vi "Read Harmonics Measure Item.vi"(0 "VISA resource name":refnum<visa-resource-name>, 5 "Harmonics Item (2: V)":u16(ring)=2 items=["Sync", "VTHD", "V", "VCON", "ATHD", "A", "ACON", "PF", "W", "WCON", "Vdeg", "Adeg"], 11 "error in (no error)":errorcluster) -> (4 "VISA resource name out":refnum<visa-resource-name>, 6 "Data":sgl[](array[numeric]) format="%^.3e", 15 "error out":errorcluster)   [LabVIEW 2013, in "Yokogawa WT200 Series.lvlib"]
doc: "This VI reads harmonic datas from the WT200 Series.\n\nNote : It needs /HRM option."
uses:
  <instrlib>/Yokogawa WT200 Series/Yokogawa WT200 Series.lvlib
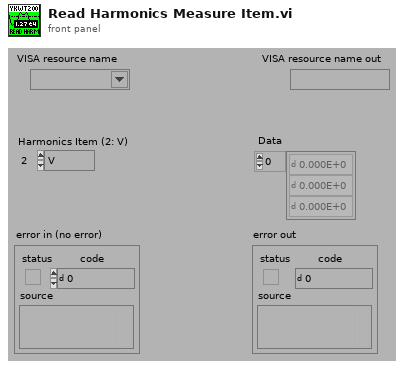
[diagram p1: front panel]
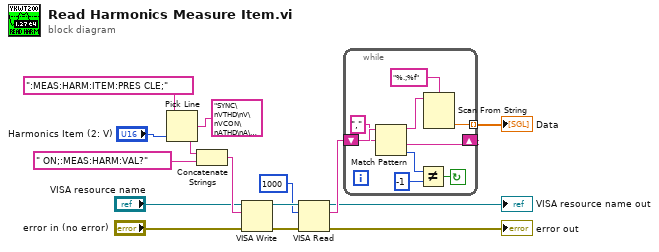
[diagram p0: block diagram]
diagram:
  n1 = Pick Line(string ("")=":MEAS:HARM:ITEM:PRES CLE;", multi-line string="SYNC\nVTHD\nV\nVCON\nATHD\nA\nACON\nPF\nW\nWCON\nVDEG\nADEG", line index="Harmonics Item (2: V)") -> (output string=w9:string)
  n2 = Concatenate Strings(w9, " ON;:MEAS:HARM:VAL?") -> (w7:string)
  n3 = VISA Write(VISA resource name="VISA resource name", write buffer=w7, error in (no error)="error in (no error)") -> (VISA resource name out=w14:refnum<visa-resource-name>, error out=w15:errorcluster)  [unwired: 1 out]
  n4 = VISA Read(VISA resource name=w14, byte count=u32 1000, error in (no error)=w15) -> (VISA resource name out=→"VISA resource name out":refnum<visa-resource-name>, read buffer=w6:string, error out=→"error out":errorcluster)  [unwired: 1 out]
  n5 = while {
    tunnel: [w17] -> w5 mode=indexing
    shift-left: w6 -> [w24]
    shift-right: [w23] -> _
    stop <- w20 continue-if-true
    n6 = Match Pattern(string=w24, regular expression=",") -> (before substring=w18:string, after substring=w23:string, offset past match=w21:i32)  [unwired: 1 in, 1 out]
    n7 = Not Equal?(x=w21, y=-1) -> (x != y?=w20:bool)
    n8 = Scan From String(format string="%.;%f", input string=w18) -> (output 1=w17:dbl)  [unwired: 3 in, 3 out]
  }
  "Data" <- w5
